vi "VeriStand FPGA DMA IO - myRIO.vi"() -> ()   [LabVIEW 2019]
uses:
  <vilib>/Platform/TimedLoop/XDataNode/wakeup.ctl
  <vilib>/Platform/TimedLoop/XDataNode/XDNodeRunTimeDep.lvlib
  <vilib>/Platform/TimedLoop/XDataNode/nitl_modes.ctl
  <vilib>/Platform/TimedLoop/XDataNode/timing_clust.ctl
  <vilib>/Platform/TimedLoop/XDataNode/XDataNode.xnode
  <vilib>/eio/EIONode/EIONode.xnode
  <vilib>/NI VeriStand/FPGA/NI_VS FPGA Support.lvlib
  <vilib>/rvi/eio/common/nirviEmuTemplateMethod_errors.vi
panel:
  in  "Generate IRQ":bool
  in  "Clock Pulse":bool
  in  "Clock Ticked":bool
  in  "Use External Timing":bool
  in  "Write to  RTSI":bool
  in  "Loop Rate (usec)":u32
  in  "Start":bool
  in  "_PWM In 1 timeout":u32=40000
  out "_PWM In 1 High Time":u32
  out "_PWM In 1 Low Time":u32
  in  "_PWM In 0 timeout":u32=40000
  out "_PWM In 0 High Time":u32
  out "_PWM In 0 Low Time":u32
  in  "_Low Pulse 3":u32
  in  "_High Pulse 3":u32
  in  "_Low Pulse 1":u32
  in  "_High Pulse 1":u32
  in  "_Low Pulse 2":u32
  in  "_High Pulse 2":u32
  in  "_Low Pulse 0":u32
  in  "_High Pulse 0":u32
  # "PWM"
  # "Configuration"
  # "Internal Controls"
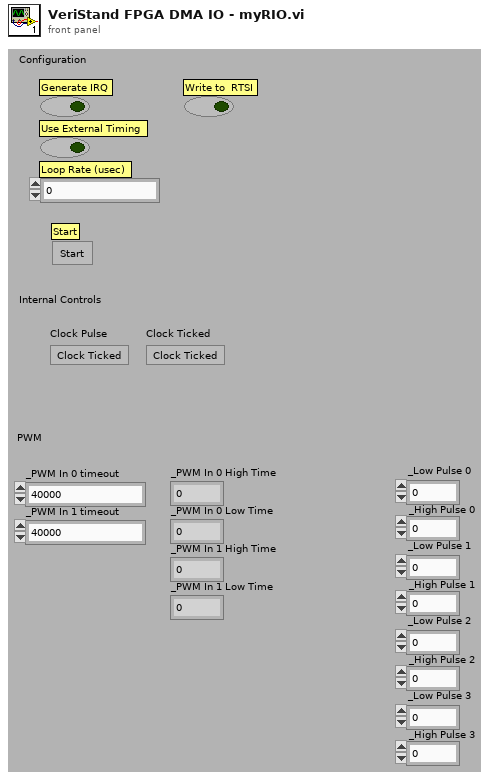
[diagram p1: front panel]
types:
  T1 = typedef "XDNodeRunTimeDep.lvlib/timing_clust.ctl" = cluster{"Expected End [f-1]":u64, "Actual End [f-1]":u64, "Finished Late? [f-1]":bool, "Expected End [i-1]":u64, "Actual End [i-1]":u64, "Finished Late? [i-1]":bool, "Expected Start [i]":u64, "Actual Start [i]":u64, "Expected Start [f]":u64, "Actual Start [f]":u64, "Source Name":string, "Structure Name":string, "Period":i64, "Deadline":i64, "Offset":i64, "Start":i64, "Priority":i32, "Timeout":i32, "Mode":T2, "Wakeup Reason":T3, "Error":errorcluster, "Source Type":string, "Secondary Source Type":string, "Global End Time":u64, "Global Start Time":u64, "Frame Duration":u64, "Iteration Duration":u64, "Assigned CPU":i32, "I/O Scan Engine Mode":u32}
  T2 = typedef "XDNodeRunTimeDep.lvlib/nitl_modes.ctl" = enum32{"No Change", "Process missed periods, maintain original phase", "Discard missed periods, maintain original phase", "Process missed periods, ignore original phase", "Discard missed periods, ignore original phase"}
  T3 = typedef "XDNodeRunTimeDep.lvlib/wakeup.ctl" = enum32{"Normal", "Aborted", "Asynchronous wakeup", "Timing source error", "Timed loop error", "Timeout"}
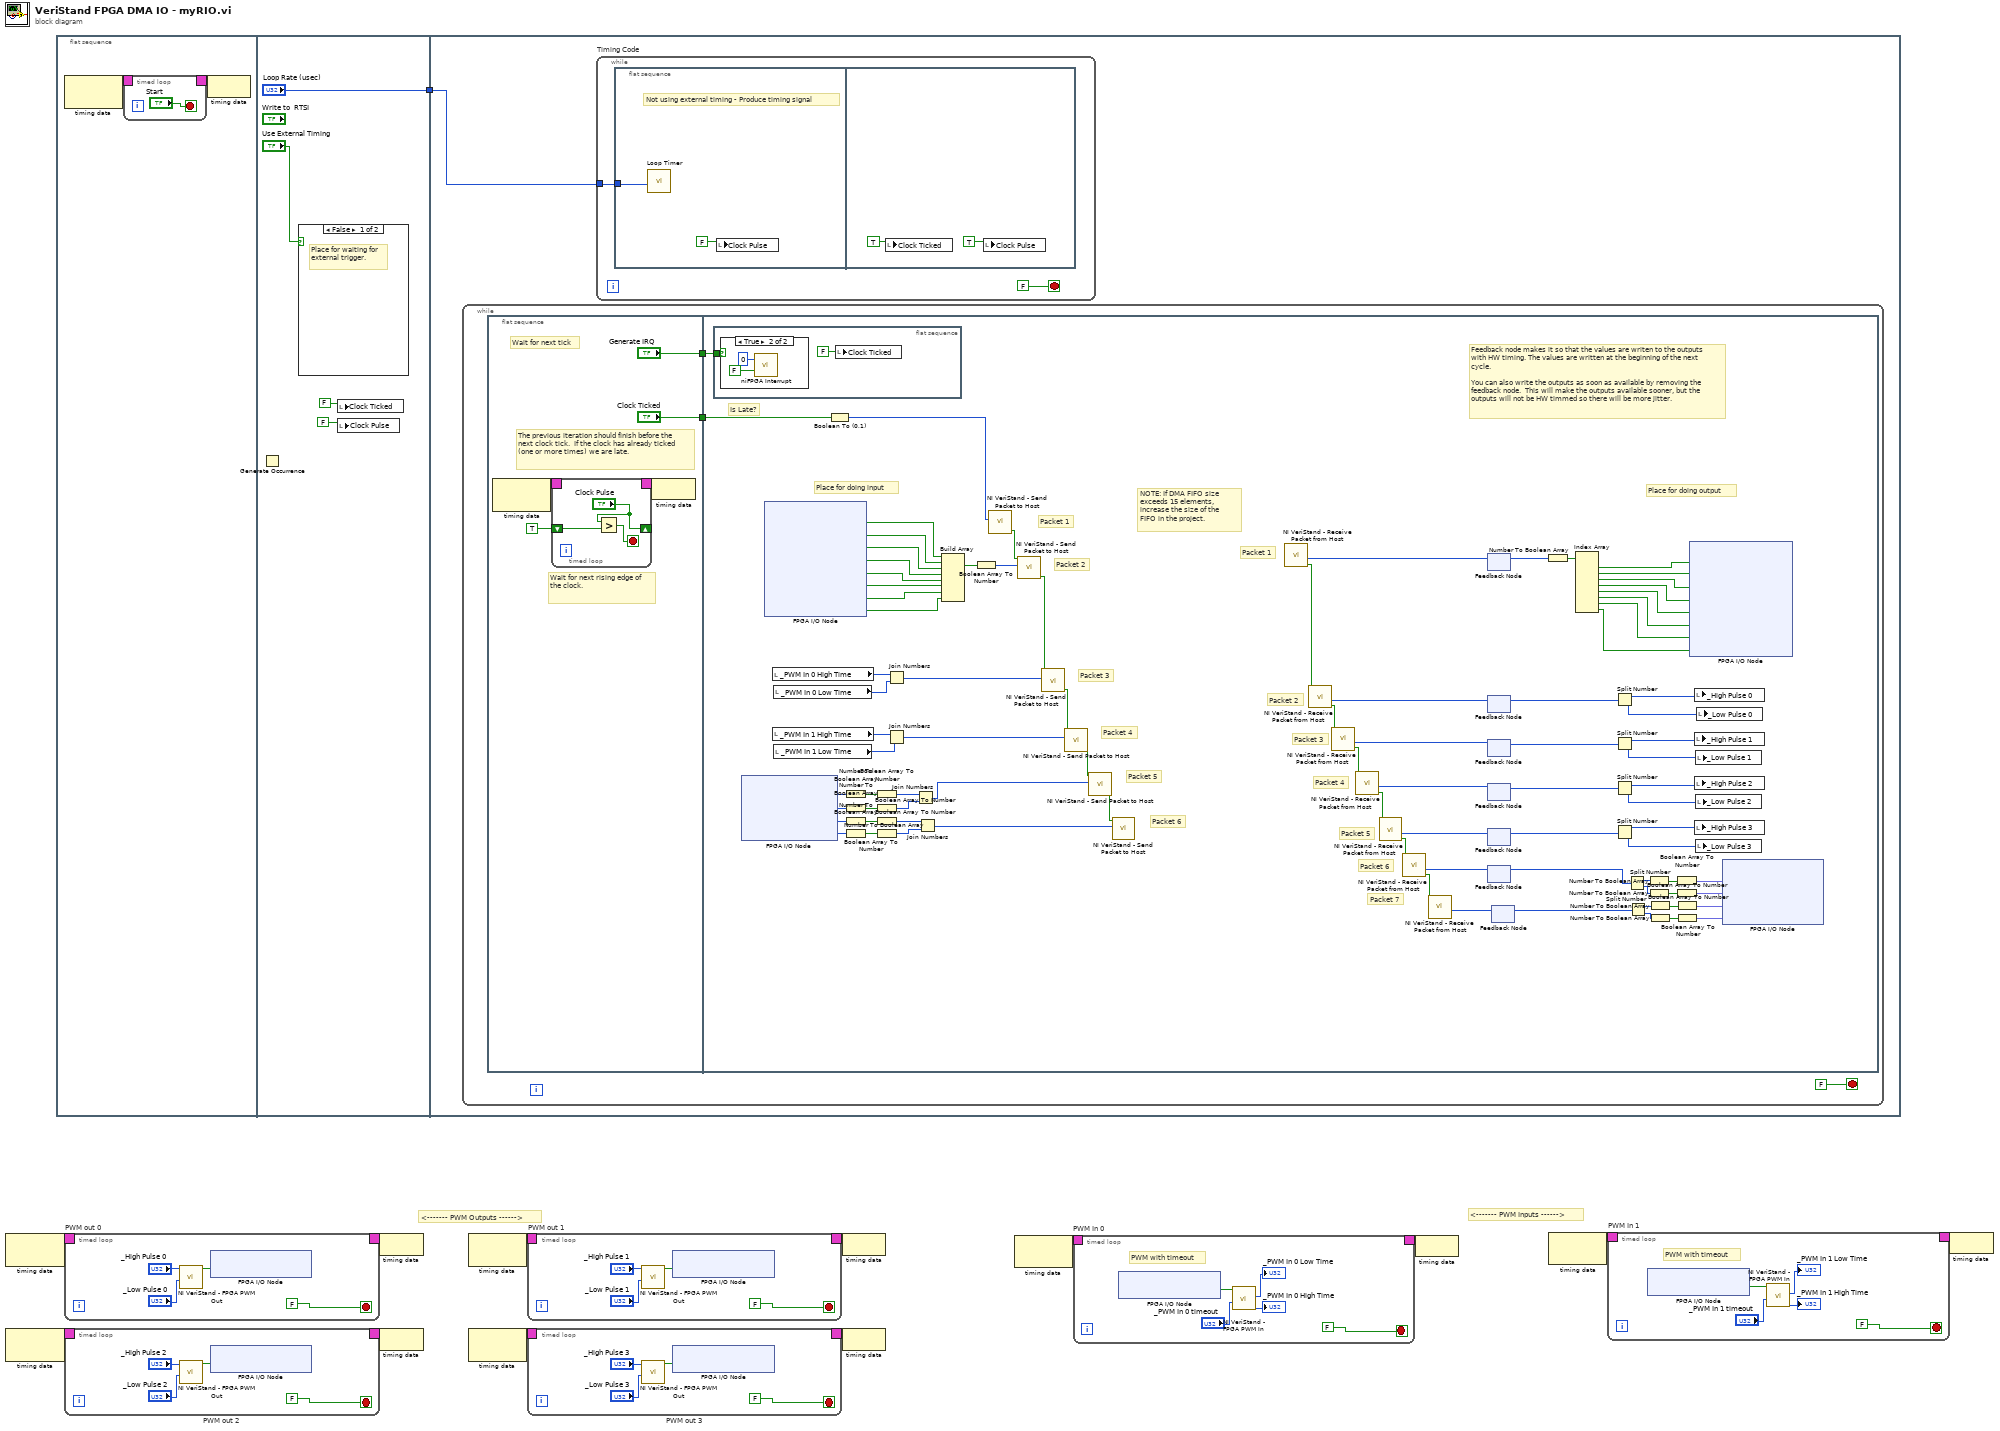
[diagram p0: block diagram]
diagram:
  # "<------- PWM Outputs ------>"
  # "<------- PWM Inputs ------>"
  n1 = node-c288() -> (w13:T1)  [unwired: 1 out]
  n2 = node-c288() -> (w11:T1)  [unwired: 1 out]
  n3 = flat-sequence {
    tunnel: ["Loop Rate (usec)"] -> w1
    tunnel: w1 -> [w25]
    frame #0 {
      n4 = node-c288() -> (w15:T1)  [unwired: 1 out]
      n5 = timed-loop {
        timing: w15 -> [_]
        timing-out: [_] -> w14
        stop <- "Start" stop-if-true
      }
      n6 = node-c288(w14) -> ()
    }
    frame #1 {
      n7 = case shown="False" "Use External Timing" {
        frame False {
          # "Place for waiting for external trigger."
        }
        frame True {
          # "Do not wait on trigger when externally timed."
        }
      }
      n8 = local write "Clock Ticked"(FALSE ("Clock Ticked")) -> ()
      n9 = local write "Clock Pulse"(FALSE ("Clock Ticked")) -> ()
    }
    frame #2 {
      n10 = while {
        stop <- FALSE stop-if-true
        n11 = flat-sequence {
          tunnel: ["Generate IRQ"] -> w33
          tunnel: ["Clock Ticked"] -> w32
          tunnel: w33 -> [w133]
          tunnel: w32 -> [w57]
          frame #0 {
            # "The previous iteration should finish before the next clock tick.  If the clock has already ticked (one or more times) we are late."
            # "Wait for next rising edge of the clock."
            # "Wait for next tick"
            n12 = node-c288() -> (w38:T1)  [unwired: 1 out]
            n13 = timed-loop {
              timing: w38 -> [_]
              timing-out: [_] -> w37
              shift-right: ["Clock Pulse"] -> _
              shift-left: TRUE ("Clock Ticked") -> [w42]
              stop <- w41 stop-if-true
              n14 = Greater?(x="Clock Pulse", y=w42) -> (0:w41:bool)
            }
            n15 = node-c288(w37) -> ()
          }
          frame #1 {
            # "Packet 6"
            # "Place for doing output"
            # "Packet 7"
            # "Packet 6"
            # "Packet 5"
            # "Packet 4"
            # "Packet 3"
            # "Packet 2"
            # "Packet 1"
            # "Packet 5"
            # "Packet 4"
            # "Packet 3"
            # "Packet 2"
            # "Packet 1"
            # "NOTE: If DMA FIFO size exceeds 15 elements, increase the size of the FIFO in the project."
            # "Is Late?"
            # "Feedback node makes it so that the values are writen to the outputs with HW timing. The values are written at the beginning of the next cycle.  \n\nYou can also write the outputs as soon as available by removing the feedback node.  This will make the outputs available sooner, but the outputs will not be HW timmed so there will be more jitter."
            # "Place for doing input"
            n16 = flat-sequence {
              tunnel: w133 -> [w135]
              frame #0 {
                n17 = case shown="True" w135 {
                  frame False {
                  }
                  frame True {
                    n18 = call <vilib>:"niFPGA Interrupt.vi"("Wait Until Cleared (F)"=FALSE ("Wait Until Cleared"), "IRQ Number (0)"=u8 0 ("IRQ Number")) -> ()  [unwired: 1 in]
                  }
                }
                n19 = local write "Clock Ticked"(FALSE ("Clock Ticked")) -> ()
              }
            }
            n20 = xnode "FPGA I/O Node"() -> ("ConnectorA/AI1"=w101:u16, "ConnectorA/AI0"=w102:u16, "ConnectorA/AI3"=w103:u16, "ConnectorA/AI2"=w104:u16)  [unwired: 4 in, 4 out]
            n21 = xnode "FPGA I/O Node"() -> ("ConnectorA/DIO0"=w113:bool, "ConnectorA/DIO1"=w114:bool, "ConnectorA/DIO2"=w115:bool, "ConnectorA/DIO3"=w116:bool, "ConnectorA/DIO4"=w54:bool, "ConnectorA/DIO5"=w53:bool, "ConnectorA/DIO6"=w52:bool, "ConnectorA/DIO7"=w51:bool)  [unwired: 8 in, 8 out]
            n22 = local read "_PWM In 0 High Time"() -> (w109:u32)
            n23 = local read "_PWM In 1 High Time"() -> (w111:u32)
            n24 = local read "_PWM In 0 Low Time"() -> (w110:u32)
            n25 = local read "_PWM In 1 Low Time"() -> (w112:u32)
            n26 = Boolean To (0,1)(Boolean=w57) -> (0, 1=w55:i16)
            n27 = Number To Boolean Array(number=w101) -> (Boolean array=w100:bool[])
            n28 = Number To Boolean Array(number=w102) -> (Boolean array=w99:bool[])
            n29 = Number To Boolean Array(number=w103) -> (Boolean array=w98:bool[])
            n30 = Number To Boolean Array(number=w104) -> (Boolean array=w97:bool[])
            n31 = Boolean Array To Number(Boolean array=w100) -> (number=w108:i32)
            n32 = Boolean Array To Number(Boolean array=w99) -> (number=w107:i32)
            n33 = Boolean Array To Number(Boolean array=w98) -> (number=w105:i32)
            n34 = Boolean Array To Number(Boolean array=w97) -> (number=w106:i32)
            n35 = Join Numbers(hi=w109, lo=w110) -> ((hi.lo)=w95:u64)
            n36 = Join Numbers(hi=w111, lo=w112) -> ((hi.lo)=w94:u64)
            n37 = Join Numbers(hi=w108, lo=w107) -> ((hi.lo)=w93:u64)
            n38 = Join Numbers(hi=w105, lo=w106) -> ((hi.lo)=w92:u64)
            n39 = Build Array(w113, w114, w115, w116, w54, w53, w52, w51) -> (w117:bool[])
            n40 = Boolean Array To Number(Boolean array=w117) -> (number=w96:u8)
            n41 = call <vilib>:"NI VeriStand - Send Packet to Host.vi"("Element"=w55) -> ("Next"=w56:bool)  [unwired: 2 in, 8 out]
            n42 = call <vilib>:"NI VeriStand - Send Packet to Host.vi"("Element"=w96, "Prev"=w56) -> ("Next"=w121:bool)  [unwired: 1 in, 8 out]
            n43 = call <vilib>:"NI VeriStand - Send Packet to Host.vi"("Element"=w95, "Prev"=w121) -> ("Next"=w120:bool)  [unwired: 1 in, 8 out]
            n44 = call <vilib>:"NI VeriStand - Send Packet to Host.vi"("Element"=w94, "Prev"=w120) -> ("Next"=w119:bool)  [unwired: 1 in, 8 out]
            n45 = call <vilib>:"NI VeriStand - Send Packet to Host.vi"("Element"=w93, "Prev"=w119) -> ("Next"=w118:bool)  [unwired: 1 in, 8 out]
            n46 = call <vilib>:"NI VeriStand - Send Packet to Host.vi"("Element"=w92, "Prev"=w118) -> ()  [unwired: 1 in, 9 out]
            n47 = call <vilib>:"NI VeriStand - Receive Packet from Host.vi"() -> ("Next"=w126:bool, "Element"=w132:u64)  [unwired: 2 in, 8 out]
            n48 = call <vilib>:"NI VeriStand - Receive Packet from Host.vi"("Prev"=w126) -> ("Next"=w125:bool, "Element"=w131:u64)  [unwired: 1 in, 8 out]
            n49 = call <vilib>:"NI VeriStand - Receive Packet from Host.vi"("Prev"=w125) -> ("Next"=w124:bool, "Element"=w130:u64)  [unwired: 1 in, 8 out]
            n50 = call <vilib>:"NI VeriStand - Receive Packet from Host.vi"("Prev"=w124) -> ("Next"=w123:bool, "Element"=w129:u64)  [unwired: 1 in, 8 out]
            n51 = call <vilib>:"NI VeriStand - Receive Packet from Host.vi"("Prev"=w123) -> ("Next"=w122:bool, "Element"=w128:u64)  [unwired: 1 in, 8 out]
            n52 = call <vilib>:"NI VeriStand - Receive Packet from Host.vi"("Prev"=w122) -> ("Next"=w59:bool, "Element"=w127:u64)  [unwired: 1 in, 8 out]
            n53 = call <vilib>:"NI VeriStand - Receive Packet from Host.vi"("Prev"=w59) -> ("Element"=w60:u64)  [unwired: 1 in, 9 out]
            n54 = feedback-in #1(w132) -> ()
            n55 = feedback #1() -> (w67:u64)  [unwired: 1 out]
            n56 = feedback-in #2(w131) -> ()
            n57 = feedback #2() -> (w66:u64)  [unwired: 1 out]
            n58 = feedback-in #3(w130) -> ()
            n59 = feedback #3() -> (w65:u64)  [unwired: 1 out]
            n60 = feedback-in #4(w129) -> ()
            n61 = feedback #4() -> (w64:u64)  [unwired: 1 out]
            n62 = feedback-in #5(w128) -> ()
            n63 = feedback #5() -> (w63:u64)  [unwired: 1 out]
            n64 = feedback-in #6(w127) -> ()
            n65 = feedback #6() -> (w62:u64)  [unwired: 1 out]
            n66 = feedback-in #7(w60) -> ()
            n67 = feedback #7() -> (w58:u64)  [unwired: 1 out]
            n68 = Number To Boolean Array(number=w67) -> (Boolean array=w87:bool[])
            n69 = Index Array(array=w87) -> (element #1=w88:bool, element #2=w89:bool, element #3=w90:bool, element #4=w91:bool, element #5=w50:bool, element #6=w49:bool, element #7=w48:bool, element #8=w47:bool)  [unwired: 8 in]
            n70 = Split Number(x=w66) -> (hi(x)=w68:u32, lo(x)=w69:u32)
            n71 = Split Number(x=w65) -> (hi(x)=w70:u32, lo(x)=w71:u32)
            n72 = Split Number(x=w64) -> (hi(x)=w72:u32, lo(x)=w73:u32)
            n73 = Split Number(x=w63) -> (hi(x)=w74:u32, lo(x)=w75:u32)
            n74 = Split Number(x=w62) -> (hi(x)=w80:u32, lo(x)=w82:u32)
            n75 = Split Number(x=w58) -> (hi(x)=w61:u32, lo(x)=w81:u32)
            n76 = Number To Boolean Array(number=w80) -> (Boolean array=w79:bool[])
            n77 = Number To Boolean Array(number=w82) -> (Boolean array=w78:bool[])
            n78 = Number To Boolean Array(number=w61) -> (Boolean array=w76:bool[])
            n79 = Number To Boolean Array(number=w81) -> (Boolean array=w77:bool[])
            n80 = Boolean Array To Number(Boolean array=w79) -> (number=w83:fxp<+/-,20,5>)
            n81 = Boolean Array To Number(Boolean array=w78) -> (number=w84:fxp<+/-,20,5>)
            n82 = Boolean Array To Number(Boolean array=w76) -> (number=w85:fxp<+/-,20,5>)
            n83 = Boolean Array To Number(Boolean array=w77) -> (number=w86:fxp<+/-,20,5>)
            n84 = xnode "FPGA I/O Node"("ConnectorC/DIO0"=w88, "ConnectorC/DIO1"=w89, "ConnectorC/DIO2"=w90, "ConnectorC/DIO3"=w91, "ConnectorC/DIO4"=w50, "ConnectorC/DIO5"=w49, "ConnectorC/DIO6"=w48, "ConnectorC/DIO7"=w47) -> ()  [unwired: 8 in, 8 out]
            n85 = local write "_High Pulse 0"(w68) -> ()
            n86 = local write "_High Pulse 1"(w70) -> ()
            n87 = local write "_High Pulse 2"(w72) -> ()
            n88 = local write "_High Pulse 3"(w74) -> ()
            n89 = local write "_Low Pulse 1"(w71) -> ()
            n90 = local write "_Low Pulse 2"(w73) -> ()
            n91 = local write "_Low Pulse 3"(w75) -> ()
            n92 = local write "_Low Pulse 0"(w69) -> ()
            n93 = xnode "FPGA I/O Node"("ConnectorA/AO1"=w83, "ConnectorA/AO0"=w84, "ConnectorB/AO1"=w85, "ConnectorB/AO0"=w86) -> ()  [unwired: 4 in, 4 out]
          }
        }
      }
      n94 = while "Timing Code" {
        tunnel: w25 -> [w27]
        stop <- FALSE stop-if-true
        n95 = flat-sequence {
          tunnel: w27 -> [w29]
          frame #0 {
            # "Not using external timing - Produce timing signal"
            n96 = call "Loop Timer"("Count(uSec)"=w29) -> ()  [unwired: 1 out]
            n97 = local write "Clock Pulse"(FALSE ("Clock Ticked")) -> ()
          }
          frame #1 {
            n98 = local write "Clock Ticked"(TRUE ("Clock Ticked")) -> ()
            n99 = local write "Clock Pulse"(TRUE ("Clock Ticked")) -> ()
          }
        }
      }
    }
  }
  n100 = timed-loop "PWM out 0" {
    timing: w13 -> [_]
    timing-out: [_] -> w12
    stop <- FALSE stop-if-true
    n101 = call <vilib>:"NI VeriStand - FPGA PWM Out.vi"("_Low Time"="_Low Pulse 0", "_High Time"="_High Pulse 0") -> ("Output"=w140:bool)  [unwired: 1 in, 8 out]
    n102 = xnode "FPGA I/O Node"("ConnectorB/DIO4"=w140) -> ()  [unwired: 1 in, 1 out]
  }
  n103 = timed-loop "PWM out 2" {
    timing: w11 -> [_]
    timing-out: [_] -> w10
    stop <- FALSE stop-if-true
    n104 = call <vilib>:"NI VeriStand - FPGA PWM Out.vi"("_Low Time"="_Low Pulse 2", "_High Time"="_High Pulse 2") -> ("Output"=w146:bool)  [unwired: 1 in, 8 out]
    n105 = xnode "FPGA I/O Node"("ConnectorB/DIO6"=w146) -> ()  [unwired: 1 in, 1 out]
  }
  n106 = Generate Occurrence() -> ()  [unwired: 1 out]
  n107 = node-c288(w12) -> ()
  n108 = node-c288(w10) -> ()
  n109 = node-c288() -> (w9:T1)  [unwired: 1 out]
  n110 = node-c288() -> (w7:T1)  [unwired: 1 out]
  n111 = timed-loop "PWM out 1" {
    timing: w9 -> [_]
    timing-out: [_] -> w8
    stop <- FALSE stop-if-true
    n112 = call <vilib>:"NI VeriStand - FPGA PWM Out.vi"("_Low Time"="_Low Pulse 1", "_High Time"="_High Pulse 1") -> ("Output"=w150:bool)  [unwired: 1 in, 8 out]
    n113 = xnode "FPGA I/O Node"("ConnectorB/DIO5"=w150) -> ()  [unwired: 1 in, 1 out]
  }
  n114 = timed-loop "PWM out 3" {
    timing: w7 -> [_]
    timing-out: [_] -> w6
    stop <- FALSE stop-if-true
    n115 = call <vilib>:"NI VeriStand - FPGA PWM Out.vi"("_Low Time"="_Low Pulse 3", "_High Time"="_High Pulse 3") -> ("Output"=w159:bool)  [unwired: 1 in, 8 out]
    n116 = xnode "FPGA I/O Node"("ConnectorB/DIO7"=w159) -> ()  [unwired: 1 in, 1 out]
  }
  n117 = node-c288(w8) -> ()
  n118 = node-c288(w6) -> ()
  n119 = node-c288() -> (w5:T1)  [unwired: 1 out]
  n120 = timed-loop "PWM In 0" {
    timing: w5 -> [_]
    timing-out: [_] -> w4
    stop <- FALSE stop-if-true
    # "PWM with timeout"
    n121 = xnode "FPGA I/O Node"() -> ("ConnectorB/DIO0"=w165:bool)  [unwired: 1 in, 1 out]
    n122 = call <vilib>:"NI VeriStand - FPGA PWM In.vi"("Time Out"="_PWM In 0 timeout", "Value"=w165) -> ("High time"=→"_PWM In 0 High Time":u32, "Low Time"=→"_PWM In 0 Low Time":u32)  [unwired: 8 out]
  }
  n123 = node-c288(w4) -> ()
  n124 = node-c288() -> (w3:T1)  [unwired: 1 out]
  n125 = timed-loop "PWM In 1" {
    timing: w3 -> [_]
    timing-out: [_] -> w2
    stop <- FALSE stop-if-true
    # "PWM with timeout"
    n126 = xnode "FPGA I/O Node"() -> ("ConnectorB/DIO1"=w172:bool)  [unwired: 1 in, 1 out]
    n127 = call <vilib>:"NI VeriStand - FPGA PWM In.vi"("Time Out"="_PWM In 1 timeout", "Value"=w172) -> ("High time"=→"_PWM In 1 High Time":u32, "Low Time"=→"_PWM In 1 Low Time":u32)  [unwired: 8 out]
  }
  n128 = node-c288(w2) -> ()
